vi "RollerPneumatic.vi"(7 "State":T1=enum."Out", 8 "Error in":errorcluster, 11 "SolenoidDevRef":T2={"DevStatus"={"status"=FALSE, "code"=0, "source"=""}, "Solenoid Module"=enum."Solenoid Module 1", "Forward Solenoid Channel"=enum."Invalid", "Reverse Solenoid Channel"=enum."Invalid"}) -> (0 "Error out":errorcluster)   [LabVIEW 2013]
doc: "VI for the clapper double solenoid. It has the following actions:\n-Init: take a reference to a double solenoid and store it in a shift register so that it does not need to be passed in again.\n-In: sets the cylinder to the in position.\n-Middle: set the cylinder to the middle position.\n-Out: set the cylinder to the out position."
uses:
  <vilib>/Rock Robotics/WPI/Solenoid/WPI_SolenoidSetEnum.vi
  <vilib>/Rock Robotics/WPI/Solenoid/WPI_SolenoidValue.ctl
  <vilib>/Rock Robotics/WPI/Solenoid/WPI_SolenoidChannel.ctl
  <vilib>/Rock Robotics/SystemInterfaces/Typedef/FPGA_TypedefSolenoidModule.ctl
  <vilib>/Rock Robotics/WPI/Solenoid/WPI_SolenoidDevRef.ctl
  DoubleSolenoidAction.ctl
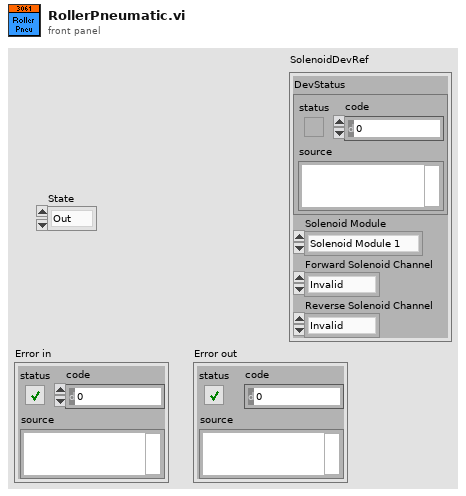
[diagram p1: front panel]
types:
  T1 = typedef "DoubleSolenoidAction.ctl" = enum16{"Init", "Middle", "In", "Out"}
  T2 = typedef "WPI_SolenoidDevRef.ctl" = cluster{"DevStatus":errorcluster, "Solenoid Module":T3, "Forward Solenoid Channel":T4, "Reverse Solenoid Channel":T4}
  T3 = typedef "FPGA_TypedefSolenoidModule.ctl" = enum16{"Solenoid Module 1", "Solenoid Module 2"}
  T4 = typedef "WPI_SolenoidChannel.ctl" = enum8{"Solenoid 1", "Solenoid 2", "Solenoid 3", "Solenoid 4", "Solenoid 5", "Solenoid 6", "Solenoid 7", "Solenoid 8", "Invalid"}
  T5 = typedef "WPI_SolenoidValue.ctl" = enum16{"Off", "On", "Forward", "Reverse"}
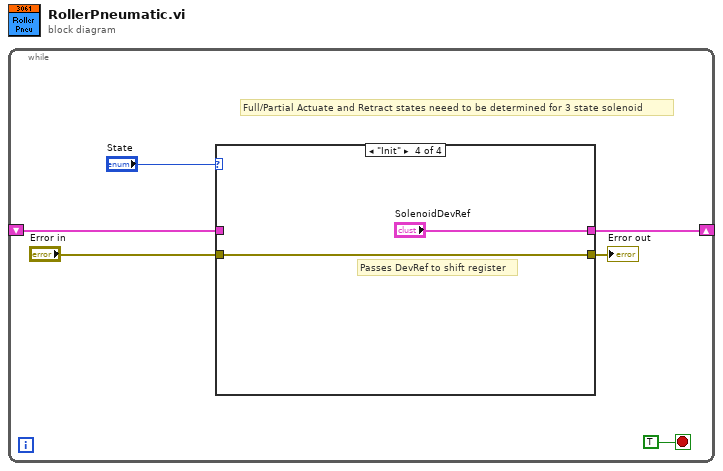
[diagram p0: block diagram]
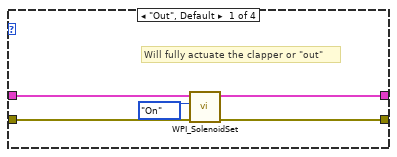
[diagram p2: hidden frame]
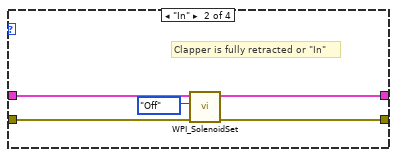
[diagram p3: hidden frame]
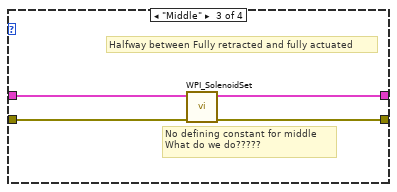
[diagram p4: hidden frame]
diagram:
  n1 = while {
    shift-right: [w4] -> _
    shift-left: _ -> [w3]
    stop <- TRUE stop-if-true
    # "Full/Partial Actuate and Retract states neeed to be determined for 3 state solenoid"
    n2 = case shown="\"Init\"" "State" {
      tunnel: [w11 w16 w20 "SolenoidDevRef"] -> w4
      tunnel: w3 -> [w9 w14 w19 _]
      tunnel: "Error in" -> [w8 w13 w18 w22]
      tunnel: [w7 w12 w17 w22] -> w1
      frame "Out", Default {
        # "Will fully actuate the clapper or \"out\""
        n3 = call-poly <vilib>:"WPI_SolenoidSet.vi"("error in (no error)"=w8, "Value"=WPI_SolenoidValue."On", "SolenoidDevRef"=w9) -> ("error out"=w7:errorcluster, "SolenoidDevRef"=w11:T2)  [unwired: 7 in]
      }
      frame "In" {
        # "Clapper is fully retracted or \"In\""
        n4 = call-poly <vilib>:"WPI_SolenoidSet.vi"("error in (no error)"=w13, "Value"=WPI_SolenoidValue."Off", "SolenoidDevRef"=w14) -> ("error out"=w12:errorcluster, "SolenoidDevRef"=w16:T2)  [unwired: 7 in]
      }
      frame "Middle" {
        # "Halfway between Fully retracted and fully actuated"
        # "No defining constant for middle\nWhat do we do?????"
        n5 = call-poly <vilib>:"WPI_SolenoidSet.vi"("error in (no error)"=w18, "SolenoidDevRef"=w19) -> ("error out"=w17:errorcluster, "SolenoidDevRef"=w20:T2)  [unwired: 8 in]
      }
      frame "Init" {
        # "Passes DevRef to shift register"
      }
    }
    "Error out" <- w1
  }
